vi "FullAlign.vi"(0 "Joystick 0":dbl, 1 "Button":bool=TRUE, 5 "Joystick 1":dbl, 7 "Distance":dbl=21.792199999999994, 9 "Angle":dbl=-43.59074216711602) -> (4 "Right Motor":dbl, 6 "Left Motor":dbl=-0.0, 10 "Not In Sight?":bool=TRUE, 15 "In Range?":bool=TRUE)   [LabVIEW 2016]
uses:
  2_11_17/Systems/Global 1.vi
panel:
  in  "MinDistance":dbl=24.0 format="%#_13g"
  out "Sees Target?":bool=TRUE
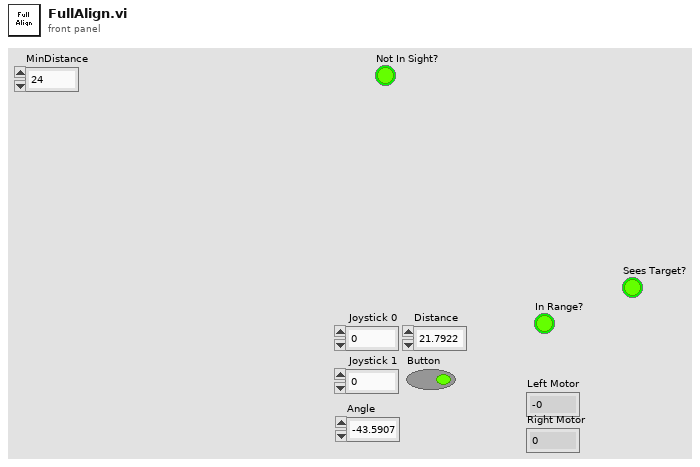
[diagram p1: front panel]
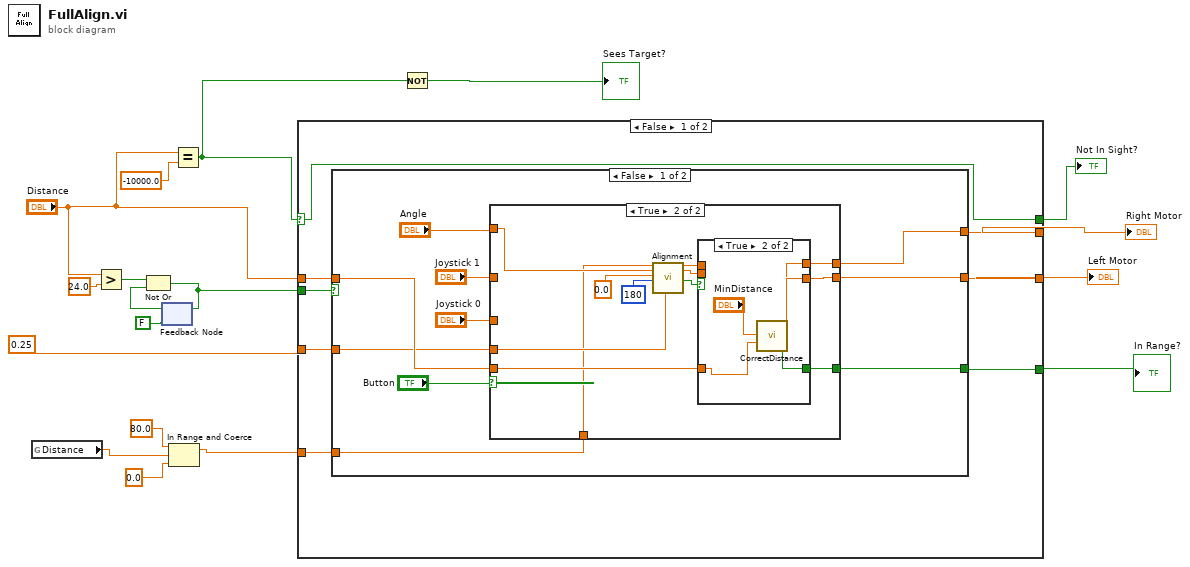
[diagram p0: block diagram]
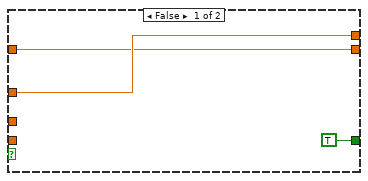
[diagram p2: hidden frame]
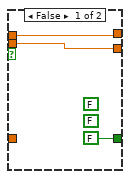
[diagram p3: hidden frame]
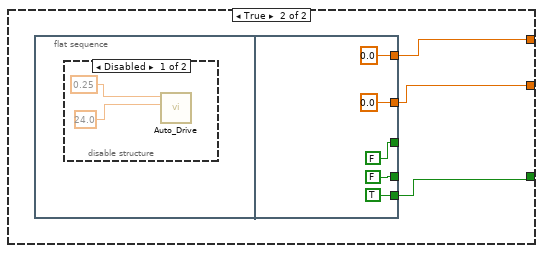
[diagram p4: hidden frame]
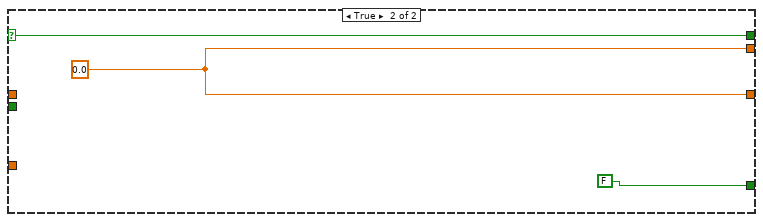
[diagram p6: hidden frame]
diagram:
  n1 = global read "Global 1.vi" "Distance"() -> (w5:dbl)
  n2 = Greater?(x="Distance", y=24.0) -> (0:w11:bool)
  n3 = feedback #1(FALSE) -> (w10:bool)
  n4 = Not Or(1:w10, 2:w11) -> (0:w12:bool)
  n5 = feedback-in #1(w12) -> ()
  n6 = In Range and Coerce(upper limit=80.0, x=w5, lower limit=0.0) -> (coerced(x)=w2:dbl)  [unwired: 1 out]
  n7 = Equal?(x="Distance", y=-10000.0) -> (x = y?=w6:bool)
  n8 = case shown="False" w6 {
    selector: w6 -> [w19 w70]
    tunnel: w12 -> [w26 _]
    tunnel: [w25 w71] -> w17
    tunnel: [w24 w71] -> w7
    tunnel: [w23 FALSE] -> w13
    tunnel: "Distance" -> [w22 _]
    tunnel: 0.25 -> [w21 _]
    tunnel: w2 -> [w20 _]
    tunnel: [w19 w70] -> w1
    frame False {
      n9 = case shown="False" w26 {
        tunnel: w22 -> [w32 _]
        tunnel: [w31 w61] -> w25
        tunnel: [w30 w60] -> w24
        tunnel: [w29 w62] -> w23
        tunnel: w21 -> [w28 _]
        tunnel: w20 -> [w27 _]
        frame False {
          n10 = case shown="True" "Button" {
            tunnel: "Joystick 1" -> [w38 _]
            tunnel: "Joystick 0" -> [w39 _]
            tunnel: [w38 w51] -> w30
            tunnel: [w39 w50] -> w31
            tunnel: "Angle" -> [_ w45]
            tunnel: [TRUE w49] -> w29
            tunnel: w32 -> [_ w48]
            tunnel: w28 -> [_ w44]
            tunnel: w27 -> [_ w40]
            frame False {
            }
            frame True {
              n11 = call "Alignment.vi"("Range"=w40, "Camera Feedback"=w45, "Target"=0.0, "POV"=180, "Turn_Gain"=w44) -> ("Right Motor"=w43:dbl, "Left Motor"=w42:dbl, "LeftAndRight?"=w41:bool)  [unwired: 12 in]
              n12 = case shown="True" w41 {
                tunnel: [w52 w58] -> w51
                tunnel: [w53 w57] -> w50
                tunnel: [FALSE w55] -> w49
                tunnel: w48 -> [_ w56]
                tunnel: w43 -> [w53 _]
                tunnel: w42 -> [w52 _]
                frame False {
                  (unwired) FALSE
                  (unwired) FALSE
                }
                frame True {
                  n13 = call "CorrectDistance.vi"("CenterPoint"="MinDistance", "Distance"=w56) -> ("In Range?"=w55:bool, "Right Motor"=w57:dbl, "Left Motor"=w58:dbl)  [unwired: 23 in]
                }
              }
            }
          }
        }
        frame True {
          n14 = flat-sequence {
            tunnel: [FALSE] -> _
            tunnel: [FALSE] -> _
            tunnel: [TRUE] -> w62
            tunnel: [0.0] -> w61
            tunnel: [0.0] -> w60
            frame #0 {
              n15 = disable-structure shown="Disabled" {
                frame Disabled {
                  n16 = call "Auto_Drive.vi"("distance"=24.0, "Drive Effort"=0.25) -> ()  [unwired: 10 in]
                }
                frame Enabled {
                }
              }
            }
            frame #1 {
            }
          }
        }
      }
    }
    frame True {
      w71 = 0.0
    }
  }
  "Right Motor" <- w17
  "Left Motor" <- w7
  "In Range?" <- w13
  "Not In Sight?" <- w1
  n17 = Not(x=w6) -> (.not. x?=→"Sees Target?":bool)
